vi "Read Contents.vi"(8 "Error in":errorcluster caption="Error in (no error)", 11 "Element Array":refnum<class "Element Array.lvclass">) -> (0 "Error out":errorcluster, 2 "Contents":refnum<class "Data Item.lvclass">[](array[class]), 3 "Element Array Out":refnum<class "Element Array.lvclass">)   [LabVIEW 2018, in "VILab.lvlib" / "Element Array.lvclass"]
uses:
  Element Array.lvclass
  Data Item.lvclass
  Element Array.lvclass/Element Array.ctl
  Attribute.lvclass
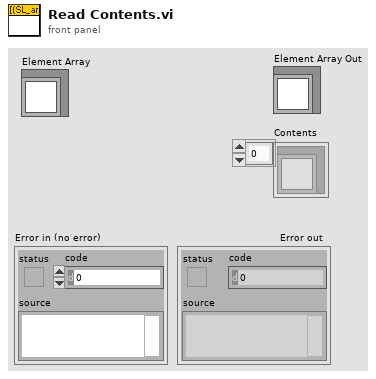
[diagram p1: front panel]
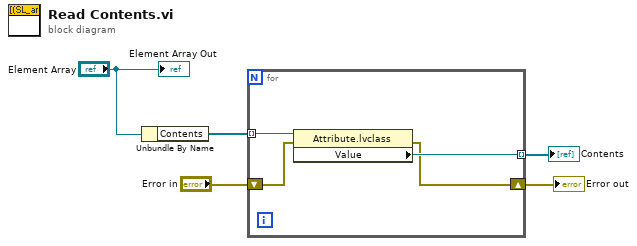
[diagram p0: block diagram]
diagram:
  n1 = Unbundle By Name("Element Array") -> ("Contents"=w4:refnum<class "Attribute.lvclass">[])
  n2 = for {
    tunnel: w4 -> [w9] mode=indexing
    shift-right: [w6] -> w1
    shift-left: "Error in" -> [w8]
    tunnel: [w7] -> w2 mode=indexing
    n3 = property class="Attribute.lvclass"(reference=w9, error in=w8) -> (error out=w6:errorcluster, "Value"=w7:refnum<class "Data Item.lvclass">)  [unwired: 1 out]
  }
  "Error out" <- w1
  "Contents" <- w2
  "Element Array Out" <- "Element Array"
